vi "Magna_custom_set_modulation_table.vi"(0 "VISA session":refnum<visa-resource-name>, 1 "Row":i8=1 min=1 max=20 step=1, 2 "Modulation Voltage":dbl min=0.0 max=2.0 format="%.3f", 3 "error in (no error)":errorcluster, 4 "Modulation Factor":dbl min=-2.0 max=1000.0 format="%.3f") -> (5 "dup VISA session":refnum<visa-resource-name>, 6 "error out":errorcluster)   [LabVIEW 2011]
doc: "This VI form sets the modulation parameters ( modulation voltage, and modulation factor) for the specified row."
uses:
  <instrlib>/mpexxx/mpexxx.llb/MPExxx Globals.gbl
panel:
  # "MAGNA-POWER"
  # "Electronics"
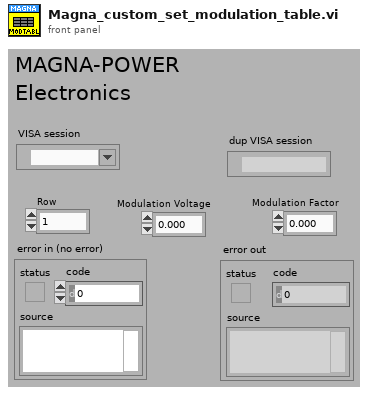
[diagram p1: front panel]
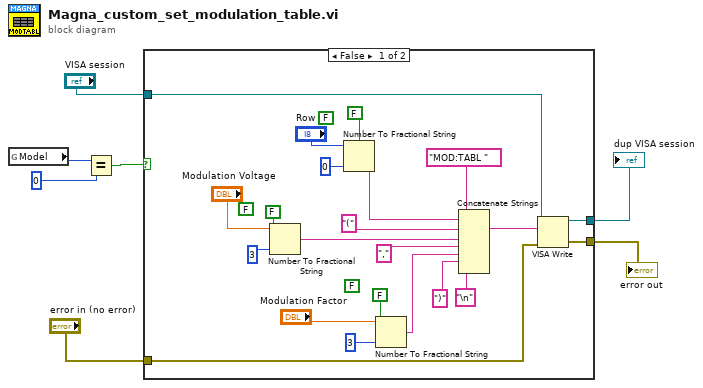
[diagram p0: block diagram]
diagram:
  n1 = global read "MPExxx Globals.gbl" "Model"() -> (w5:u8)
  n2 = Equal?(x=w5, y=0) -> (x = y?=w7:bool)
  n3 = case shown="False" w7 {
    tunnel: "VISA session" -> [w14 w31]
    tunnel: "error in (no error)" -> [w13 w30]
    tunnel: [w12 w30] -> w2
    tunnel: [w11 w31] -> w1
    frame False {
      (unwired) FALSE ("use system decimal point (T)")
      (unwired) FALSE ("use system decimal point (T)")
      (unwired) FALSE ("use system decimal point (T)")
      n4 = Number To Fractional String(use system decimal point (T)=FALSE, number="Modulation Voltage", precision (6)=3) -> (F-format string=w17:string)  [unwired: 1 in]
      n5 = Number To Fractional String(use system decimal point (T)=FALSE, number="Row", precision (6)=0) -> (F-format string=w18:string)  [unwired: 1 in]
      n6 = Number To Fractional String(use system decimal point (T)=FALSE, number="Modulation Factor", precision (6)=3) -> (F-format string=w16:string)  [unwired: 1 in]
      n7 = Concatenate Strings("MOD:TABL ", w18, "(", w17, ",", w16, ")", "\n") -> (w15:string)
      n8 = VISA Write(VISA resource name=w14, write buffer=w15, error in (no error)=w13) -> (VISA resource name out=w11:refnum<visa-resource-name>, error out=w12:errorcluster)  [unwired: 1 out]
    }
    frame True {
    }
  }
  "error out" <- w2
  "dup VISA session" <- w1
